vi "Alarm.vi"(0 "Alarm M10":bool[](array[boolean]), 2 "Alarm M1":bool[](array[boolean]), 4 "Alarm S10":bool[](array[boolean]), 5 "Alarm S1":bool[](array[boolean]), 7 "Second Ones":bool[](array[boolean]), 9 "Second Tens":bool[](array[boolean]), 11 "Minute Ones":bool[](array[boolean]), 13 "Minute Tens":bool[](array[boolean])) -> (16 "Alarm":bool)   [LabVIEW 2014]
panel:
  # "Alarm Set"
  # "Clock Input"
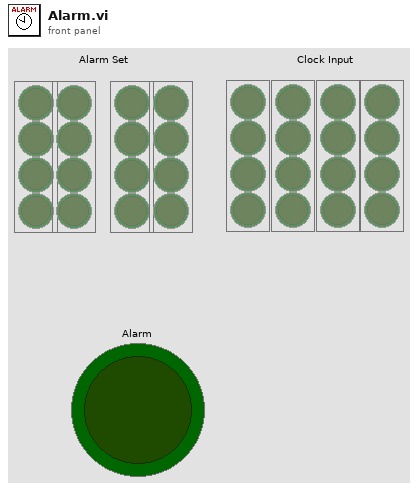
[diagram p1: front panel]
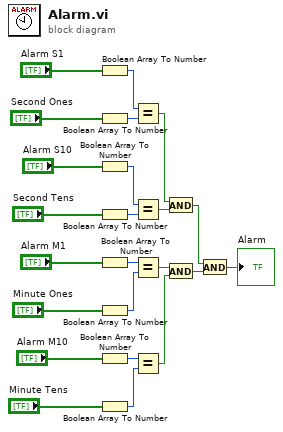
[diagram p0: block diagram]
diagram:
  n1 = Boolean Array To Number(Boolean array="Alarm S1") -> (number=w22:u32)
  n2 = Boolean Array To Number(Boolean array="Second Ones") -> (number=w21:u32)
  n3 = Boolean Array To Number(Boolean array="Alarm S10") -> (number=w19:u32)
  n4 = Boolean Array To Number(Boolean array="Second Tens") -> (number=w20:u32)
  n5 = Boolean Array To Number(Boolean array="Alarm M1") -> (number=w18:u32)
  n6 = Boolean Array To Number(Boolean array="Minute Ones") -> (number=w17:u32)
  n7 = Boolean Array To Number(Boolean array="Alarm M10") -> (number=w15:u32)
  n8 = Boolean Array To Number(Boolean array="Minute Tens") -> (number=w16:u32)
  n9 = Equal?(x=w22, y=w21) -> (x = y?=w9:bool)
  n10 = Equal?(x=w19, y=w20) -> (x = y?=w8:bool)
  n11 = Equal?(x=w18, y=w17) -> (x = y?=w7:bool)
  n12 = Equal?(x=w15, y=w16) -> (x = y?=w6:bool)
  n13 = And(x=w9, y=w8) -> (x .and. y?=w10:bool)
  n14 = And(x=w7, y=w6) -> (x .and. y?=w11:bool)
  n15 = And(x=w10, y=w11) -> (x .and. y?=→"Alarm":bool)
